vi "Util U8 Bytes to U16.vi"(8 "error in (no error)":errorcluster) -> (0 "error out":errorcluster)   [LabVIEW 2017, in "xHelper.lvlib"]
uses:
  xHelper.lvlib
panel:
  in  "index":i32
  out "U16":u16
  in  "U8 Array":u8[](array[numeric]) format="%x"
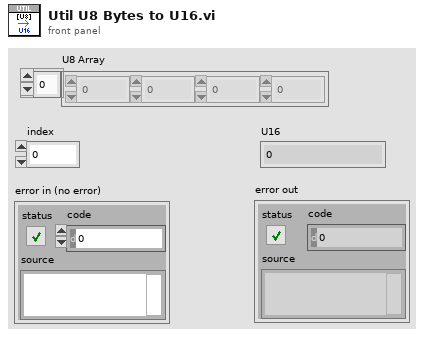
[diagram p1: front panel]
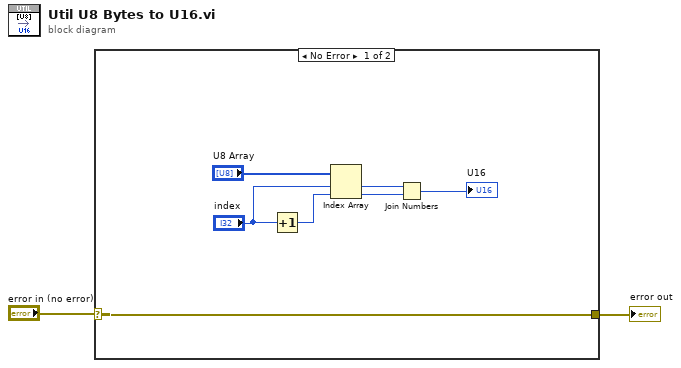
[diagram p0: block diagram]
diagram:
  n1 = case shown="No Error" "error in (no error)" {
    selector: "error in (no error)" -> [w3 w10]
    tunnel: [w3 w10] -> w1
    frame No Error {
      n2 = Increment(x="index") -> (x+1=w7:i32)
      n3 = Index Array(array="U8 Array", index #1="index", index #2=w7) -> (element #1=w6:u8, element #2=w5:u8)
      n4 = Join Numbers(hi=w6, lo=w5) -> ((hi.lo)=→"U16":u16)
    }
    frame Error {
    }
  }
  "error out" <- w1
